vi "Read Response Status.vi"(8 "error in (no error)":errorcluster, 11 "HttpResponseMessage in":refnum<class "HttpResponseMessage.lvclass">) -> (0 "error out":errorcluster, 1 "ReasonPhrase":string, 2 "StatusCode":i32(ring)=100 items=["Continue"=100, "SwitchingProtocols"=101, "OK"=200, "Created"=201, "Accepted"=202, "NonAuthoritativeInformation"=203, "NoContent"=204, "ResetContent"=205, "PartialContent"=206, "MultipleChoices, Ambiguous"=300, "MovedPermanently, Moved"=301, "Found, Redirect"=302, "SeeOther, RedirectMethod"=303, "NotModified"=304, "UseProxy"=305, "Unused"=306, "TemporaryRedirect, RedirectKeepVerb"=307, "BadRequest"=400, "Unauthorized"=401, "PaymentRequired"=402, "Forbidden"=403, "NotFound"=404, "MethodNotAllowed"=405, "NotAcceptable"=406, "ProxyAuthenticationRequired"=407, "RequestTimeout"=408, "Conflict"=409, "Gone"=410, "LengthRequired"=411, "PreconditionFailed"=412, "RequestEntityTooLarge"=413, "RequestUriTooLong"=414, "UnsupportedMediaType"=415, "RequestedRangeNotSatisfiable"=416, "ExpectationFailed"=417, "UpgradeRequired"=426, "InternalServerError"=500, "NotImplemented"=501, "BadGateway"=502, "ServiceUnavailable"=503, "GatewayTimeout"=504, "HttpVersionNotSupported"=505], 3 "HttpResponseMessage out":refnum<class "HttpResponseMessage.lvclass">, 4 "IsSuccessStatusCode":bool, 5 "StatusCode_num":i32)   [LabVIEW 2018, in "HttpClient_NET.lvlib" / "HttpResponseMessage.lvclass"]
doc: "<b> </b> <b> </b>\nHttpClient_NET\nJustin Young - Viviota\nCopyright (c) 2021\nLicense: BSD"
uses:
  HttpResponseMessage.lvclass
  HttpResponseMessage.lvclass/HttpResponseMessage.ctl
  Accessors/Read NET_HttpReponseMessage.vi
  System.Net.Http
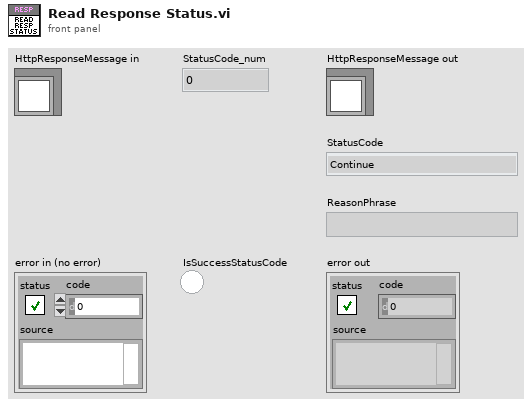
[diagram p1: front panel]
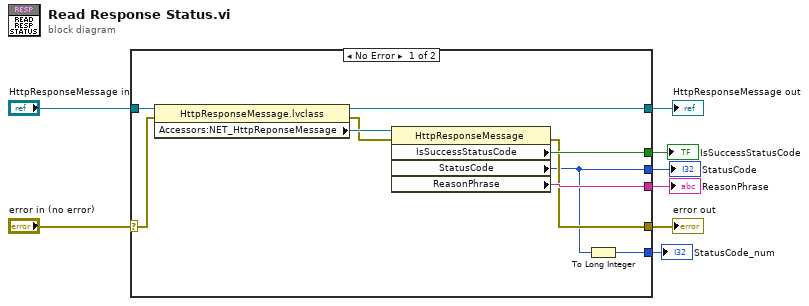
[diagram p0: block diagram]
diagram:
  n1 = case shown="No Error" "error in (no error)" {
    selector: "error in (no error)" -> [w18 w20]
    tunnel: [w11 w20] -> w7
    tunnel: [w16 w19] -> w5
    tunnel: "HttpResponseMessage in" -> [w17 w19]
    tunnel: [w14 _] -> w4
    tunnel: [w10 _] -> w3
    tunnel: [w13 _] -> w2
    tunnel: [w9 _] -> w1
    frame No Error {
      n2 = property class="HttpResponseMessage.lvclass"(reference=w17, error in=w18) -> (reference out=w16:refnum<class "HttpResponseMessage.lvclass">, error out=w12:errorcluster, "Accessors:NET_HttpReponseMessage"=w15:refnum<k24>)
      n3 = property class="HttpResponseMessage"(reference=w15, error in=w12) -> (error out=w11:errorcluster, "IsSuccessStatusCode"=w13:bool, "StatusCode"=w10:i32, "ReasonPhrase"=w14:string)  [unwired: 1 out]
      n4 = To Long Integer(number=w10) -> (32bit integer=w9:i32)
    }
    frame Error {
    }
  }
  "error out" <- w7
  "HttpResponseMessage out" <- w5
  "IsSuccessStatusCode" <- w2
  "StatusCode" <- w3
  "ReasonPhrase" <- w4
  "StatusCode_num" <- w1
